vi "Run Action_Do.vi"(8 "error in (no error)":errorcluster, 10 "Project Builder in":refnum<class "Project Builder.lvclass">, 11 "Report":refnum<class "Report Action.lvclass">) -> (0 "error out":errorcluster, 1 "Success?":bool, 3 "Report":refnum<class "Report Data.lvclass">)   [LabVIEW 2020, in "ProjectBuilder.lvlib" / "Report Action.lvclass"]
uses:
  Report Action.lvclass
  Project Builder/Project Builder.lvclass
  Data/Report Data/Report Data.lvclass
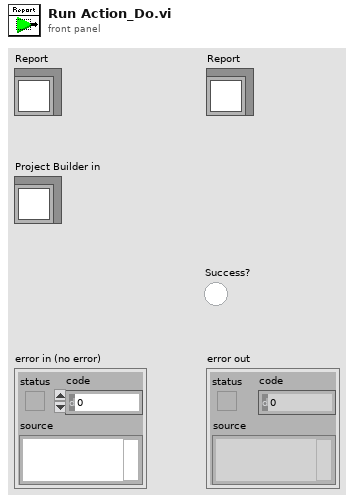
[diagram p1: front panel]
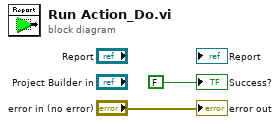
[diagram p0: block diagram]
diagram:
  "error out" <- "error in (no error)"
  "Success?" <- FALSE
